vi "Lab Panel V6.00.vi"() -> ()   [LabVIEW 2017] (continued)
                n3701 = Greater?(x=w6518, y=w6517) -> (0:w6516:bool)
                n3702 = case shown="True" w6516 {
                  frame False {
                  }
                  frame True {
                    n3703 = local read "ON L05-2"() -> (w6520:cluster{"amps":dbl, "volts":dbl, "pf":dbl})
                    n3704 = global write "Global display 2.vi" "ON L05-2"(w6520) -> ()
                  }
                }
              }
            }
            n3705 = global write "Global display 3.vi" "TEMP RS 05-2"(w6377) -> ()
            n3706 = global write "Global display 3.vi" "TEMP RS 05-1"(w6378) -> ()
            n3707 = global write "Global display 3.vi" "TEMP RS 03-2"(w6381) -> ()
            n3708 = global write "Global display 3.vi" "TEMP RS 02-1"(w6384) -> ()
            n3709 = global write "Global display 3.vi" "TEMP RS 02-2"(w6383) -> ()
            n3710 = global write "Global display 3.vi" "TEMP RS 04-2"(w6379) -> ()
            n3711 = global write "Global display 3.vi" "TEMP RS 01-2"(w6385) -> ()
            n3712 = global write "Global display 3.vi" "TEMP RS 03-1"(w6382) -> ()
            n3713 = global write "Global display 3.vi" "TEMP RS 04-1"(w6380) -> ()
            n3714 = global write "Global display 3.vi" "TEMP RS 01-1"(w6386) -> ()
            n3715 = global write "Global display 2.vi" "RESULT LAB05-1"(w6422) -> ()
            n3716 = global write "Global display 2.vi" "RESULT LAB01-2"(w6429) -> ()
            n3717 = global write "Global display 2.vi" "RESULT LAB03-2"(w6425) -> ()
            n3718 = global write "Global display 2.vi" "RESULT LAB04-1"(w6424) -> ()
            n3719 = global write "Global display 2.vi" "RESULT LAB04-2"(w6423) -> ()
            n3720 = global write "Global display 2.vi" "RESULT LAB05-2"(w6421) -> ()
            n3721 = global write "Global display 2.vi" "RESULT LAB03-1"(w6426) -> ()
            n3722 = global write "Global display 2.vi" "RESULT LAB01-1"(w6430) -> ()
            n3723 = global write "Global display 2.vi" "RESULT LAB02-1"(w6428) -> ()
            n3724 = global write "Global display 2.vi" "RESULT LAB02-2"(w6427) -> ()
          }
          frame #23 {
            # "simulate values"
            n3725 = global write "Global display 4.vi" "LAB deg C"("LAB deg C") -> ()
          }
          frame #24 {
            # "end main and display program"
            n3726 = stacked-sequence {
              seq-local: [_ w6527 _] -> [_ _ w6534]
              tunnel: w6523 -> [w6524 _ _]
              tunnel: w6522 -> [_ _ w6532]
              frame #0 {
                n3727 = case shown="True" w6524 {
                  frame False {
                  }
                  frame True {
                    n3728 = One Button Dialog(message="Excessive number of USB \nresets done, re-start program.") -> ()  [unwired: 1 in, 1 out]
                  }
                }
              }
              frame #1 {
                # "check for reset error"
                n3729 = local read "DAQ Simulate"() -> (w6526:bool)
                n3730 = case shown="False" w6526 {
                  tunnel: [w6528 FALSE] -> w6527
                  frame False {
                    n3731 = local read "Reset Error"() -> (w6528:bool)
                    n3732 = case shown="True" w6528 {
                      frame False {
                      }
                      frame True {
                        n3733 = One Button Dialog(message="USB ERROR, program will be stopped.\nClose program, close windows, switch panel off\nand re power panel. If error persists seek help.") -> ()  [unwired: 1 in, 1 out]
                      }
                    }
                  }
                  frame True {
                  }
                }
              }
              frame #2 {
                # "end labview session"
                n3734 = case shown="True" w6532 {
                  tunnel: [_ TRUE] -> w6531
                  frame False {
                  }
                  frame True {
                    n3735 = call "sub vi - AI USB4704 (3)  Close Task v2.vi"() -> ()  [unwired: 16 in]
                  }
                }
                n3736 = Or(x=w6534, y="stop all") -> (x .or. y?=w6533:bool)
                n3737 = case shown="True" w6533 {
                  tunnel: w6531 -> [_ _]
                  frame False {
                  }
                  frame True {
                    n3738 = stacked-sequence {
                      frame #0 {
                        n3739 = global write "Global display 1.vi" "stop disp"(TRUE) -> ()
                      }
                      frame #1 {
                        n3740 = call "sub vi - AI USB4704 (3)  Close Task v2.vi"() -> ()  [unwired: 16 in]
                      }
                      frame #2 {
                        n3741 = Quit LabVIEW(quit? (T)=TRUE) -> ()
                      }
                    }
                  }
                }
              }
            }
          }
          frame #25 {
            n3742 = disable-structure shown="Enabled" {
              disable-tunnel: [w6549 _] -> w6539
              frame Disabled {
                n3743 = call <userlib>:"Periodic Trigger__ogtk.vi"("time (ms)"=u32 750) -> ("Triggered"=w6549:bool)  [unwired: 12 in, 2 out]
                n3744 = case shown="True" w6549 {
                  frame False {
                  }
                  frame True {
                    n3745 = local read "Application Directory"() -> (w6551:path)
                    n3746 = control-ref of="This VI"() -> (w6560:refnum<vi>)
                    n3747 = control-ref of="Main Control"() -> (w6558:refnum<vi>)
                    n3748 = Bundle By Name(cluster=T25 {"Tab Ref"=refnum, "Values"=[]} ("Image Data"), "Tab Ref"=w6558, "Values"=i32[] [0, 2]) -> (w6556:T25)
                    n3749 = call "SaveWWWImages2.vi"("Image Data 2"=w6556, "Destination"=w6551, "VI in"=w6560) -> ()  [unwired: 9 in]
                    n3750 = control-ref of="LAB01 deg C"() -> (w6553:refnum<vi>)
                    n3751 = control-ref of="LAB01 AMPS"() -> (w6555:refnum<vi>)
                    n3752 = control-ref of="LAB01 VOLTS"() -> (w6554:refnum<vi>)
                    n3753 = Build Array(w6555, w6554, w6553) -> (w6552:refnum<vi>[])
                    n3754 = call "SaveWWWChartImages.vi"("Chart Refs"=w6552, "Destination"=w6551) -> ()  [unwired: 10 in]
                  }
                }
              }
              frame Enabled {
              }
            }
            n3755 = disable-structure shown="Enabled" {
              disable-tunnel: w6539 -> [w6540 _]
              frame Disabled {
                n3756 = case shown="False" w6540 {
                  frame False {
                    n3757 = call <userlib>:"Periodic Trigger__ogtk.vi"("time (ms)"=u32 2000) -> ("Triggered"=w6541:bool)  [unwired: 12 in, 2 out]
                    n3758 = case shown="True" w6541 {
                      frame False {
                      }
                      frame True {
                        n3759 = local read "Application Directory"() -> (w6544:path)
                        n3760 = control-ref of="This VI"() -> (w6545:refnum<vi>)
                        n3761 = control-ref of="Main Control"() -> (w6543:refnum<vi>)
                        n3762 = Bundle By Name(cluster=T25 {"Tab Ref"=refnum, "Values"=[]} ("Image Data"), "Tab Ref"=w6543, "Values"=i32[] [1, 5]) -> (w6546:T25)
                        n3763 = call "SaveWWWImages2.vi"("Image Data 2"=w6546, "Destination"=w6544, "VI in"=w6545) -> ()  [unwired: 9 in]
                      }
                    }
                  }
                  frame True {
                  }
                }
              }
              frame Enabled {
              }
            }
          }
          frame #26 {
            n3764 = Tick Count (ms)() -> (millisecond timer value=w6563:u32)
            n3765 = Subtract(x=w6563, y=w6562) -> (x-y=→"Loop Time":u32)
          }
        }
        n3766 = node-c288() -> ()  [unwired: 1 in, 1 out]
        "loops" <- w386
      }
      n3767 = node-c288(w356) -> ()  [unwired: 1 out]
    }
  }
